vi "mainActivity_关闭日志服务.vi"(8 "错误输入（无错误）":errorcluster) -> (0 "错误输出":errorcluster)   [LabVIEW 2014]
uses:
  R/manifest.vi
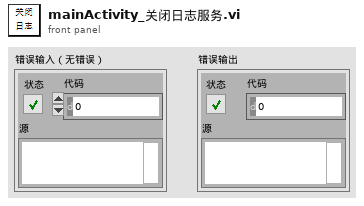
[diagram p1: front panel]
types:
  T1 = cluster{"标题":string, "相对路径":string, "类型":enum16{"服务", "活动"}, "专属队列名称":string}
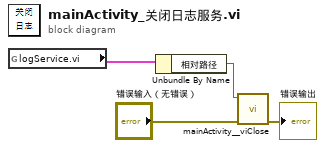
[diagram p0: block diagram]
diagram:
  n1 = global read "manifest.vi" "logService.vi"() -> (w2:T1)
  n2 = Unbundle By Name(w2) -> ("相对路径"=w1:string)
  n3 = call "mainActivity__viClose.vi"("error in"="错误输入（无错误）", "urlStr"=w1) -> ("error out"=→"错误输出":errorcluster)  [unwired: 8 in, 1 out]
